vi "Load from file.vi"(8 "error in (no error)":errorcluster, 10 "file path (use dialog)":path, 11 "UserPwd DB in":refnum<class "UserPwd DB.lvclass">) -> (0 "error out":errorcluster, 3 "UserPwd DB out":refnum<class "UserPwd DB.lvclass">)   [LabVIEW 2016, in "UserPwd DB.lvlib" / "UserPwd DB.lvclass"]
uses:
  <userlib>/Common Components/UserPwd DB/UserPwd DB/UserPwd DB.lvclass
  <userlib>/Common Components/UserPwd DB/UserPwd DB/UserPwd DB.lvclass/UserPwd DB.ctl
  <vilib>/addons/_JKI.lib/Serialization/JSON/JKI JSON Serialization.lvlib
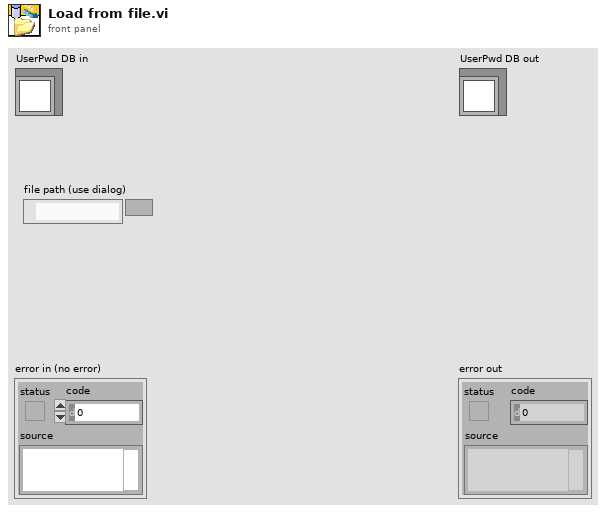
[diagram p1: front panel]
types:
  T1 = enum16{"open", "replace", "create", "open or create", "replace or create", "replace or create with confirmation"}
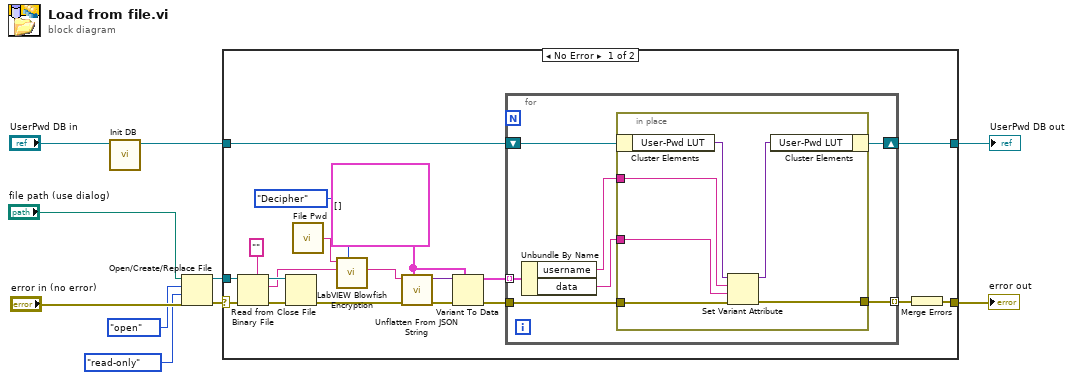
[diagram p0: block diagram]
diagram:
  n1 = call <userlib>:"Init DB.vi"("UserPwd DB in"="UserPwd DB in") -> ("UserPwd DB out"=w1:refnum<class "UserPwd DB.lvclass">)  [unwired: 9 in, 1 out]
  n2 = Open/Create/Replace File(file path (use dialog)="file path (use dialog)", error in="error in (no error)", operation (0:open)=T1."open", access (0:read/write)=enum16{"read/write", "read-only", "write-only"}."read-only") -> (refnum out=w6:refnum<file>, error out=w4:errorcluster)  [unwired: 2 in, 1 out]
  n3 = case shown="No Error" w4 {
    selector: w4 -> [w25 w44]
    tunnel: w6 -> [w28 _]
    tunnel: [w17 w44] -> w5
    tunnel: w1 -> [w15 w43]
    tunnel: [w14 w43] -> w2
    frame No Error {
      w20 = cluster{"username":string, "data":string}[] [] ("Array")
      n4 = Read from Binary File(5:"", 8:w25, 11:w28) -> (0:w29:errorcluster, 2:w22:string, 3:w26:refnum<file>)  [unwired: 3 in, 1 out]
      n5 = Close File(refnum=w26, error in=w29) -> (error out=w27:errorcluster)  [unwired: 1 out]
      n6 = call <userlib>:"File Pwd.vi"() -> ("String"=w12:string)
      n7 = call <userlib>:"LabVIEW Blowfish Encryption.vi"("Password"=w12, "Enc/Dec"=enum16{"Encipher", "Decipher"}."Decipher", "Input Text"=w22) -> ("Output text"=w13:string)  [unwired: 3 in, 2 out]
      n8 = call <vilib>:"Unflatten From JSON String.vi"("Type and Defaults"=w20, "error in (no error)"=w27, "JSON String"=w13) -> ("error out"=w23:errorcluster, "Variant"=w21:variant)  [unwired: 7 in]
      n9 = Variant To Data(error in=w23, type=w20, Variant=w21) -> (data=w16:cluster{"username":string, "data":string}[], error out=w19:errorcluster)
      n10 = for {
        tunnel: w19 -> [w31]
        tunnel: [w30] -> w18 mode=indexing
        tunnel: w16 -> [w36] mode=indexing
        shift-right: [w34] -> w14
        shift-left: w15 -> [w35]
        n11 = Unbundle By Name(w36) -> ("username"=w33:string, "data"=w32:string)
        n12 = in-place {
          in-place-border: w33 -> [w40]
          in-place-border: w32 -> [w39]
          in-place-border: [w38] -> w30
          in-place-border: w31 -> [w37]
          n13 = in-place-cluster #1(w35) -> ("User-Pwd LUT"=w42:variant)
          n14 = Set Variant Attribute(Variant=w42, name=w40, value=w39, error in=w37) -> (Variant out=w41:variant, error out=w38:errorcluster)  [unwired: 1 out]
          n15 = in-place-cluster #1("User-Pwd LUT"=w41) -> (w34:refnum<class "UserPwd DB.lvclass">)
        }
      }
      n16 = Merge Errors(w18) -> (w17:errorcluster)
    }
    frame Error {
    }
  }
  "error out" <- w5
  "UserPwd DB out" <- w2
